vi "SubtractU8Baseline.vi"(8 "Cutoff U8":u8, 10 "Baseline U8":u8, 11 "Analog data cluster in":T1) -> (2 "Over? Array":bool[](array[boolean]), 3 "Analog data cluster out":T1)   [LabVIEW 2014]
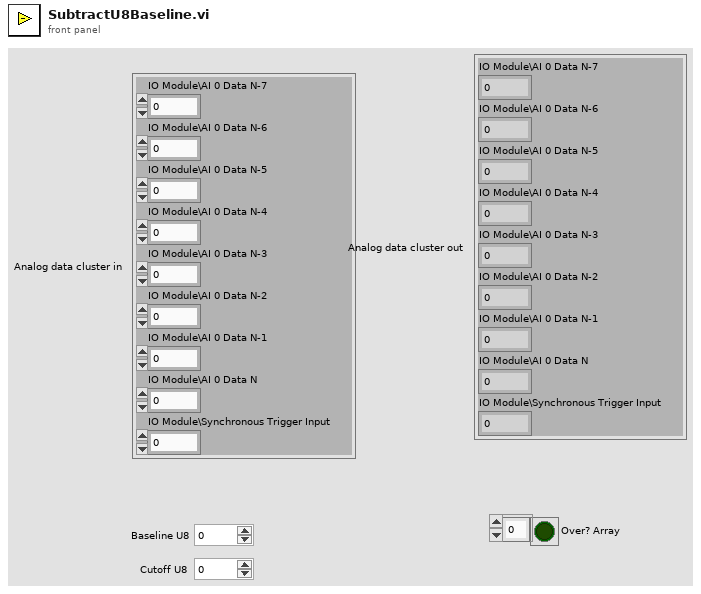
[diagram p1: front panel]
types:
  T1 = cluster{"IO Module\\AI 0 Data N-7":u8, "IO Module\\AI 0 Data N-6":u8, "IO Module\\AI 0 Data N-5":u8, "IO Module\\AI 0 Data N-4":u8, "IO Module\\AI 0 Data N-3":u8, "IO Module\\AI 0 Data N-2":u8, "IO Module\\AI 0 Data N-1":u8, "IO Module\\AI 0 Data N":u8, "IO Module\\Synchronous Trigger Input":u8}
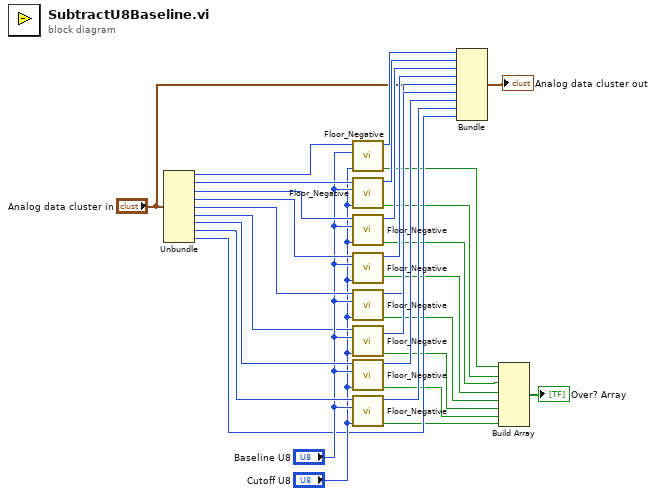
[diagram p0: block diagram]
diagram:
  n1 = Unbundle("Analog data cluster in") -> ("IO Module\\AI 0 Data N-7"=w21:u8, "IO Module\\AI 0 Data N-6"=w15:u8, "IO Module\\AI 0 Data N-5"=w16:u8, "IO Module\\AI 0 Data N-4"=w17:u8, "IO Module\\AI 0 Data N-3"=w18:u8, "IO Module\\AI 0 Data N-2"=w13:u8, "IO Module\\AI 0 Data N-1"=w19:u8, "IO Module\\AI 0 Data N"=w20:u8, "IO Module\\Synchronous Trigger Input"=w10:u8)
  n2 = call "Floor_Negative.vi"("Cutoff U8"="Cutoff U8", "Baseline U8"="Baseline U8", "Input Value"=w21) -> ("Over?"=w9:bool, "Output Value"=w29:u8)  [unwired: 7 in]
  n3 = call "Floor_Negative.vi"("Cutoff U8"="Cutoff U8", "Baseline U8"="Baseline U8", "Input Value"=w15) -> ("Over?"=w2:bool, "Output Value"=w22:u8)  [unwired: 7 in]
  n4 = call "Floor_Negative.vi"("Cutoff U8"="Cutoff U8", "Baseline U8"="Baseline U8", "Input Value"=w16) -> ("Over?"=w3:bool, "Output Value"=w23:u8)  [unwired: 7 in]
  n5 = call "Floor_Negative.vi"("Cutoff U8"="Cutoff U8", "Baseline U8"="Baseline U8", "Input Value"=w17) -> ("Over?"=w4:bool, "Output Value"=w24:u8)  [unwired: 7 in]
  n6 = call "Floor_Negative.vi"("Cutoff U8"="Cutoff U8", "Baseline U8"="Baseline U8", "Input Value"=w18) -> ("Over?"=w5:bool, "Output Value"=w25:u8)  [unwired: 7 in]
  n7 = call "Floor_Negative.vi"("Cutoff U8"="Cutoff U8", "Baseline U8"="Baseline U8", "Input Value"=w13) -> ("Over?"=w6:bool, "Output Value"=w26:u8)  [unwired: 7 in]
  n8 = call "Floor_Negative.vi"("Cutoff U8"="Cutoff U8", "Baseline U8"="Baseline U8", "Input Value"=w19) -> ("Over?"=w7:bool, "Output Value"=w27:u8)  [unwired: 7 in]
  n9 = call "Floor_Negative.vi"("Cutoff U8"="Cutoff U8", "Baseline U8"="Baseline U8", "Input Value"=w20) -> ("Over?"=w8:bool, "Output Value"=w28:u8)  [unwired: 7 in]
  n10 = Bundle(cluster="Analog data cluster in", "IO Module\\AI 0 Data N-7"=w29, "IO Module\\AI 0 Data N-6"=w22, "IO Module\\AI 0 Data N-5"=w23, "IO Module\\AI 0 Data N-4"=w24, "IO Module\\AI 0 Data N-3"=w25, "IO Module\\AI 0 Data N-2"=w26, "IO Module\\AI 0 Data N-1"=w27, "IO Module\\AI 0 Data N"=w28, "IO Module\\Synchronous Trigger Input"=w10) -> (→"Analog data cluster out":T1)
  n11 = Build Array(w9, w2, w3, w4, w5, w6, w7, w8) -> (→"Over? Array":bool[])
